vi "Rename Any Implemented Method.vi"(8 "error in":errorcluster, 9 "Name":string, 10 "Class To Rename":refnum<vi>) -> (0 "error out":errorcluster)   [LabVIEW 2021, in "_Rename.lvlib"]
uses:
  _Rename.lvlib
  <vilib>/Utility/traverseref.llb/TRef TravTarget.ctl
  <vilib>/Utility/traverseref.llb/VI Scripting - Traverse.lvlib
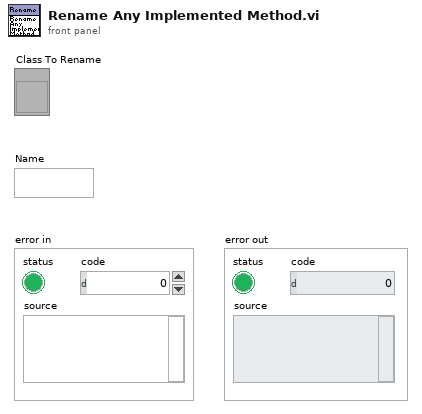
[diagram p1: front panel]
types:
  T1 = typedef "TRef TravTarget.ctl" = enum16{"FP", "BD", "Other"}
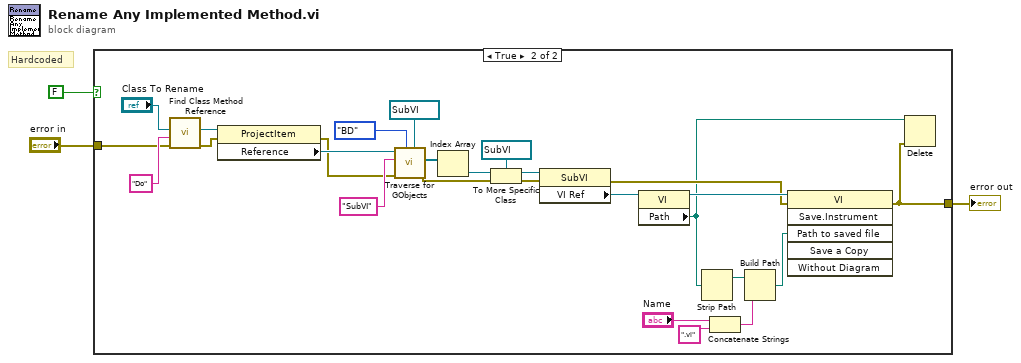
[diagram p0: block diagram]
diagram:
  # "Hardcoded"
  n1 = case shown="True" FALSE {
    tunnel: "error in" -> [w4 w7]
    tunnel: [w4 w13] -> w3
    frame False {
    }
    frame True {
      n2 = call "Find Class Method Reference.vi"("error in"=w7, "Method Name"="Do" ("regular expression"), "Class Reference"="Class To Rename") -> ("error out"=w5:errorcluster, "Method Reference"=w6:refnum<vi>)  [unwired: 7 in]
      n3 = property class="ProjectItem"(reference=w6, error in=w5) -> (error out=w14:errorcluster, "Reference"=w15:refnum<vi>)  [unwired: 1 out]
      n4 = call <vilib>:"Traverse for GObjects.vi"("Other Refnum"=refnum<vi> refnum, "Traverse Target"=TRef_TravTarget."BD", "error in (no error)"=w14, "Class Name"="SubVI", "VI Refnum"=w15) -> ("error out"=w28:errorcluster, "References"=w27:refnum<vi>[])  [unwired: 3 in, 2 out]
      n5 = Index Array(array=w27) -> (element=w25:refnum<vi>)  [unwired: 1 in]
      n6 = To More Specific Class(target class=refnum<vi> refnum ("Other Refnum"), reference=w25, error in=w28) -> (specific class reference=w24:refnum<vi>, error out=w26:errorcluster)
      n7 = property class="SubVI"(reference=w24, error in=w26) -> (error out=w18:errorcluster, "VI Ref"=w22:refnum<vi>)  [unwired: 1 out]
      n8 = property class="VI"(reference=w22) -> (reference out=w21:refnum<vi>, "Path"=w12:path)  [unwired: 1 in, 1 out]
      n9 = Strip Path(path=w12) -> (stripped path=w20:path)  [unwired: 1 out]
      n10 = Concatenate Strings("Name", ".vi" ("string")) -> (w16:string)
      n11 = Build Path(base path=w20, name or relative path=w16) -> (appended path=w19:path)
      n12 = invoke class="VI" method="Save.Instrument"(reference=w21, error in=w18, "Path to saved file"=w19) -> (error out=w13:errorcluster)  [unwired: 3 in, 5 out]
      n13 = Delete(path (use dialog)=w12, error in=w13) -> ()  [unwired: 3 in, 3 out]
    }
  }
  "error out" <- w3
